vi "Motion Profile Generator Jerk Limited.vi"() -> ()   [LabVIEW 2016]
panel:
  out "Final Position":dbl=202.3936431884765
  out "acceleration rotations/sec^2":dbl[](array[numeric])=[0.0, 2.2612551610354346, 4.522510322070869, 6.783765483106304, 9.045020644141736, 11.30627580517718, 13.567530966212601, 15.828786127248051, 18.090041288283476, 20.351296449318905, 22.612551610354323, 24.873806771389795, 27.135061932425213, 29.396317093460667, 31.657572254496067, 33.91882741553147, 36.18008257656694, 38.441337737602375, 40.702592898637846, 42.96384805967321, 45.22510322070865, 47.48635838174408, 49.74761354277966, 52.008868703814954, 54.27012386485039, 56.531379025885826, 58.79263418692133, 58.79263418692119, 56.531379025885826, 54.27012386485046, 52.0088687038151, 49.74761354277945, 47.48635838174408, 45.22510322070886, 42.96384805967321, 40.702592898637704, 38.44133773760234, 36.180082576567116, 33.918827415531325, 31.657572254496245, 29.396317093460596, 27.13506193242523, 24.873806771389866, 22.612551610354217, 20.351296449319136, 18.090041288283203, 15.828786127248122, 13.567530966212757, 11.306275805177393, 9.045020644141744, 6.7837654831060945, 4.522510322071014, 0.0, -4.522510322071014, -6.7837654831060945, -9.045020644141744, -11.306275805177393, -13.567530966212473, -15.828786127248122, -18.090041288283203, -20.351296449319136, -22.612551610353933, -24.87380677139015, -27.135061932424946, -29.39631709346088, -31.65757225449596, -33.91882741553161, -36.18008257656669, -38.44133773760248, -40.70259289863799, -42.96384805967307, -45.22510322070872, -47.48635838174408, -49.74761354277959, -52.00886870381467, -54.2701238648506, -56.531379025885826, -58.792634186921475, -58.79263418692119, -56.531379025885684, -54.27012386485046, -52.008868703815025, -49.74761354277952, -47.486358381744154, -45.22510322070872, -42.96384805967335, -40.702592898637775, -38.44133773760241, -36.18008257656694, -33.91882741553154, -31.657572254496102, -29.396317093460667, -27.13506193242525, -24.873806771389813, -22.61255161035436, -20.351296449318923, -18.090041288283523, -15.82878612724806, -13.567530966212637, -11.306275805177197, -9.04502064414177, -6.783765483106331, -4.522510322070896, -2.261255161035462, -2.774099786489076e-14]
  out "Position rotations":dbl[](array[numeric])=[0.0, 0.002826568951294293, 0.014132844756471467, 0.039571965318120114, 0.08479706853882882, 0.15546129232118616, 0.2572177745677807, 0.3957196531812011, 0.5766200660640359, 0.8055721511188737, 1.088229046248303, 1.4302438893549125, 1.8372698183412908, 2.314959971110026, 2.8689674855637075, 3.5049454996049234, 4.2285471511362624, 5.045425578060313, 5.961233918279664, 6.981625309696904, 8.11225289021462, 9.358769797735404, 10.72682917016184, 12.222084145396522, 13.850187861342034, 15.616793455900966, 17.52755406697591, 19.585296263518153, 21.787193476576405, 24.12759256824808, 26.600840400630585, 29.201283835821336, 31.92326973591774, 34.76114496301721, 37.70925637921716, 40.761950846614994, 43.91357522730813, 47.158476383393975, 50.491001176969945, 53.90549647013345, 57.396309124981904, 60.95778600361271, 64.58427396812328, 68.27011988061105, 72.00967060317339, 75.79727299790774, 79.6272739269115, 83.4940202522821, 87.39185883611692, 91.31513654051341, 95.25820022756895, 99.21539675938097, 103.17824642909557, 107.13544296090758, 111.07850664796312, 115.0017843523596, 118.89962293619443, 122.76636926156503, 126.5963701905688, 130.38397258530316, 134.1235233078655, 137.80936922035326, 141.43585718486383, 144.99733406349463, 148.48814671834307, 151.90264201150657, 155.23516680508254, 158.4800679611684, 161.63169234186154, 164.68438680925937, 167.6324982254593, 170.47037345255876, 173.19235935265516, 175.79280278784591, 178.2660506202284, 180.6064497119001, 182.80834692495836, 184.8660891215006, 186.77684973257556, 188.5434553271345, 190.17155904308, 191.66681401831468, 193.03487339074113, 194.2813902982619, 195.4120178787796, 196.43240927019684, 197.34821761041619, 198.16509603734025, 198.8886976888716, 199.52467570291282, 200.0786832173665, 200.55637337013522, 200.9633992991216, 201.3054141422282, 201.58807103735762, 201.81702312241245, 201.99792353529529, 202.1364254139087, 202.2381818961553, 202.30884611993767, 202.35407122315837, 202.37951034372003, 202.3908166195252, 202.3936431884765, 202.3936431884765]
  out "velocity rotations/sec":dbl[](array[numeric])=[0.0, 0.11306275805177173, 0.3391882741553152, 0.6783765483106304, 1.1306275805177173, 1.6959413707765763, 2.3743179190872064, 3.165757225449609, 4.070259289863783, 5.087824112329728, 6.218451692847444, 7.462142031416934, 8.818895128038195, 10.288710982711228, 11.871589595436031, 13.567530966212605, 15.376535095040952, 17.29860198192107, 19.333731626852963, 21.481924029836623, 23.743179190872056, 26.11749710995926, 28.604877787098243, 31.20532122228899, 33.91882741553151, 36.7453963668258, 39.68502807617187, 42.62465978551793, 45.45122873681222, 48.16473493005474, 50.7651783652455, 53.25255904238447, 55.62687696147167, 57.888132122507116, 60.03632452549078, 62.07145417042266, 63.99352105730278, 65.80252518613113, 67.4984665569077, 69.08134516963251, 70.55116102430554, 71.9079141209268, 73.1516044594963, 74.28223204001401, 75.29979686247997, 76.20429892689413, 76.99573823325653, 77.67411478156717, 78.23942857182604, 78.69167960403313, 79.03086787818843, 79.25699339429198, 79.25699339429198, 79.03086787818843, 78.69167960403313, 78.23942857182604, 77.67411478156717, 76.99573823325655, 76.20429892689414, 75.29979686247998, 74.28223204001402, 73.15160445949633, 71.90791412092682, 70.55116102430557, 69.08134516963253, 67.49846655690773, 65.80252518613115, 63.993521057302814, 62.07145417042269, 60.03632452549079, 57.88813212250714, 55.6268769614717, 53.2525590423845, 50.76517836524552, 48.164734930054784, 45.451228736812254, 42.62465978551796, 39.68502807617189, 36.74539636682583, 33.918827415531545, 31.205321222289022, 28.60487778709827, 26.117497109959295, 23.743179190872088, 21.48192402983665, 19.333731626852984, 17.298601981921095, 15.376535095040975, 13.567530966212628, 11.87158959543605, 10.288710982711246, 8.818895128038212, 7.46214203141695, 6.218451692847459, 5.087824112329741, 4.070259289863795, 3.165757225449619, 2.374317919087216, 1.6959413707765842, 1.1306275805177244, 0.6783765483106359, 0.3391882741553193, 0.1130627580517745, 1.3870498932445381e-15, 0.0]
  out "XY Graph":cluster{dbl[], dbl[]}[](graph)=[{[0.0, 0.05, 0.1, 0.15000000000000002, 0.2, 0.25, 0.30000000000000004, 0.35000000000000003, 0.4, 0.45, 0.5, 0.55, 0.6000000000000001, 0.65, 0.7000000000000001, 0.75, 0.8, 0.8500000000000001, 0.9, 0.9500000000000001, 1.0, 1.05, 1.1, 1.1500000000000001, 1.2000000000000002, 1.25, 1.3, 1.35, 1.4000000000000001, 1.4500000000000002, 1.5, 1.55, 1.6, 1.6500000000000001, 1.7000000000000002, 1.75, 1.8, 1.85, 1.9000000000000001, 1.9500000000000002, 2.0, 2.0500000000000003, 2.1, 2.15, 2.2, 2.25, 2.3000000000000003, 2.35, 2.4000000000000004, 2.45, 2.5, 2.5500000000000003, 2.6, 2.6500000000000004, 2.7, 2.75, 2.8000000000000003, 2.85, 2.9000000000000004, 2.95, 3.0, 3.0500000000000003, 3.1, 3.1500000000000004, 3.2, 3.25, 3.3000000000000003, 3.35, 3.4000000000000004, 3.45, 3.5, 3.5500000000000003, 3.6, 3.6500000000000004, 3.7, 3.75, 3.8000000000000003, 3.85, 3.9000000000000004, 3.95, 4.0, 4.05, 4.1000000000000005, 4.15, 4.2, 4.25, 4.3, 4.3500000000000005, 4.4, 4.45, 4.5, 4.55, 4.6000000000000005, 4.65, 4.7, 4.75, 4.800000000000001, 4.8500000000000005, 4.9, 4.95, 5.0, 5.050000000000001, 5.1000000000000005, 5.15, 5.2], [0.0, 0.11306275805177173, 0.3391882741553152, 0.6783765483106304, 1.1306275805177173, 1.6959413707765763, 2.3743179190872064, 3.165757225449609, 4.070259289863783, 5.087824112329728, 6.218451692847444, 7.462142031416934, 8.818895128038195, 10.288710982711228, 11.871589595436031, 13.567530966212605, 15.376535095040952, 17.29860198192107, 19.333731626852963, 21.481924029836623, 23.743179190872056, 26.11749710995926, 28.604877787098243, 31.20532122228899, 33.91882741553151, 36.7453963668258, 39.68502807617187, 42.62465978551793, 45.45122873681222, 48.16473493005474, 50.7651783652455, 53.25255904238447, 55.62687696147167, 57.888132122507116, 60.03632452549078, 62.07145417042266, 63.99352105730278, 65.80252518613113, 67.4984665569077, 69.08134516963251, 70.55116102430554, 71.9079141209268, 73.1516044594963, 74.28223204001401, 75.29979686247997, 76.20429892689413, 76.99573823325653, 77.67411478156717, 78.23942857182604, 78.69167960403313, 79.03086787818843, 79.25699339429198, 79.25699339429198, 79.03086787818843, 78.69167960403313, 78.23942857182604, 77.67411478156717, 76.99573823325655, 76.20429892689414, 75.29979686247998, 74.28223204001402, 73.15160445949633, 71.90791412092682, 70.55116102430557, 69.08134516963253, 67.49846655690773, 65.80252518613115, 63.993521057302814, 62.07145417042269, 60.03632452549079, 57.88813212250714, 55.6268769614717, 53.2525590423845, 50.76517836524552, 48.164734930054784, 45.451228736812254, 42.62465978551796, 39.68502807617189, 36.74539636682583, 33.918827415531545, 31.205321222289022, 28.60487778709827, 26.117497109959295, 23.743179190872088, 21.48192402983665, 19.333731626852984, 17.298601981921095, 15.376535095040975, 13.567530966212628, 11.87158959543605, 10.288710982711246, 8.818895128038212, 7.46214203141695, 6.218451692847459, 5.087824112329741, 4.070259289863795, 3.165757225449619, 2.374317919087216, 1.6959413707765842, 1.1306275805177244, 0.6783765483106359, 0.3391882741553193, 0.1130627580517745, 1.3870498932445381e-15, 0.0]}, {[0.0, 0.05, 0.1, 0.15000000000000002, 0.2, 0.25, 0.30000000000000004, 0.35000000000000003, 0.4, 0.45, 0.5, 0.55, 0.6000000000000001, 0.65, 0.7000000000000001, 0.75, 0.8, 0.8500000000000001, 0.9, 0.9500000000000001, 1.0, 1.05, 1.1, 1.1500000000000001, 1.2000000000000002, 1.25, 1.3, 1.35, 1.4000000000000001, 1.4500000000000002, 1.5, 1.55, 1.6, 1.6500000000000001, 1.7000000000000002, 1.75, 1.8, 1.85, 1.9000000000000001, 1.9500000000000002, 2.0, 2.0500000000000003, 2.1, 2.15, 2.2, 2.25, 2.3000000000000003, 2.35, 2.4000000000000004, 2.45, 2.5, 2.5500000000000003, 2.6, 2.6500000000000004, 2.7, 2.75, 2.8000000000000003, 2.85, 2.9000000000000004, 2.95, 3.0, 3.0500000000000003, 3.1, 3.1500000000000004, 3.2, 3.25, 3.3000000000000003, 3.35, 3.4000000000000004, 3.45, 3.5, 3.5500000000000003, 3.6, 3.6500000000000004, 3.7, 3.75, 3.8000000000000003, 3.85, 3.9000000000000004, 3.95, 4.0, 4.05, 4.1000000000000005, 4.15, 4.2, 4.25, 4.3, 4.3500000000000005, 4.4, 4.45, 4.5, 4.55, 4.6000000000000005, 4.65, 4.7, 4.75, 4.800000000000001, 4.8500000000000005, 4.9, 4.95, 5.0, 5.050000000000001, 5.1000000000000005, 5.15, 5.2], [0.0, 0.002826568951294293, 0.014132844756471467, 0.039571965318120114, 0.08479706853882882, 0.15546129232118616, 0.2572177745677807, 0.3957196531812011, 0.5766200660640359, 0.8055721511188737, 1.088229046248303, 1.4302438893549125, 1.8372698183412908, 2.314959971110026, 2.8689674855637075, 3.5049454996049234, 4.2285471511362624, 5.045425578060313, 5.961233918279664, 6.981625309696904, 8.11225289021462, 9.358769797735404, 10.72682917016184, 12.222084145396522, 13.850187861342034, 15.616793455900966, 17.52755406697591, 19.585296263518153, 21.787193476576405, 24.12759256824808, 26.600840400630585, 29.201283835821336, 31.92326973591774, 34.76114496301721, 37.70925637921716, 40.761950846614994, 43.91357522730813, 47.158476383393975, 50.491001176969945, 53.90549647013345, 57.396309124981904, 60.95778600361271, 64.58427396812328, 68.27011988061105, 72.00967060317339, 75.79727299790774, 79.6272739269115, 83.4940202522821, 87.39185883611692, 91.31513654051341, 95.25820022756895, 99.21539675938097, 103.17824642909557, 107.13544296090758, 111.07850664796312, 115.0017843523596, 118.89962293619443, 122.76636926156503, 126.5963701905688, 130.38397258530316, 134.1235233078655, 137.80936922035326, 141.43585718486383, 144.99733406349463, 148.48814671834307, 151.90264201150657, 155.23516680508254, 158.4800679611684, 161.63169234186154, 164.68438680925937, 167.6324982254593, 170.47037345255876, 173.19235935265516, 175.79280278784591, 178.2660506202284, 180.6064497119001, 182.80834692495836, 184.8660891215006, 186.77684973257556, 188.5434553271345, 190.17155904308, 191.66681401831468, 193.03487339074113, 194.2813902982619, 195.4120178787796, 196.43240927019684, 197.34821761041619, 198.16509603734025, 198.8886976888716, 199.52467570291282, 200.0786832173665, 200.55637337013522, 200.9633992991216, 201.3054141422282, 201.58807103735762, 201.81702312241245, 201.99792353529529, 202.1364254139087, 202.2381818961553, 202.30884611993767, 202.35407122315837, 202.37951034372003, 202.3908166195252, 202.3936431884765, 202.3936431884765]}, {[0.0, 0.05, 0.1, 0.15000000000000002, 0.2, 0.25, 0.30000000000000004, 0.35000000000000003, 0.4, 0.45, 0.5, 0.55, 0.6000000000000001, 0.65, 0.7000000000000001, 0.75, 0.8, 0.8500000000000001, 0.9, 0.9500000000000001, 1.0, 1.05, 1.1, 1.1500000000000001, 1.2000000000000002, 1.25, 1.3, 1.35, 1.4000000000000001, 1.4500000000000002, 1.5, 1.55, 1.6, 1.6500000000000001, 1.7000000000000002, 1.75, 1.8, 1.85, 1.9000000000000001, 1.9500000000000002, 2.0, 2.0500000000000003, 2.1, 2.15, 2.2, 2.25, 2.3000000000000003, 2.35, 2.4000000000000004, 2.45, 2.5, 2.5500000000000003, 2.6, 2.6500000000000004, 2.7, 2.75, 2.8000000000000003, 2.85, 2.9000000000000004, 2.95, 3.0, 3.0500000000000003, 3.1, 3.1500000000000004, 3.2, 3.25, 3.3000000000000003, 3.35, 3.4000000000000004, 3.45, 3.5, 3.5500000000000003, 3.6, 3.6500000000000004, 3.7, 3.75, 3.8000000000000003, 3.85, 3.9000000000000004, 3.95, 4.0, 4.05, 4.1000000000000005, 4.15, 4.2, 4.25, 4.3, 4.3500000000000005, 4.4, 4.45, 4.5, 4.55, 4.6000000000000005, 4.65, 4.7, 4.75, 4.800000000000001, 4.8500000000000005, 4.9, 4.95, 5.0, 5.050000000000001, 5.1000000000000005, 5.15, 5.2], [0.0, 2.2612551610354346, 4.522510322070869, 6.783765483106304, 9.045020644141736, 11.30627580517718, 13.567530966212601, 15.828786127248051, 18.090041288283476, 20.351296449318905, 22.612551610354323, 24.873806771389795, 27.135061932425213, 29.396317093460667, 31.657572254496067, 33.91882741553147, 36.18008257656694, 38.441337737602375, 40.702592898637846, 42.96384805967321, 45.22510322070865, 47.48635838174408, 49.74761354277966, 52.008868703814954, 54.27012386485039, 56.531379025885826, 58.79263418692133, 58.79263418692119, 56.531379025885826, 54.27012386485046, 52.0088687038151, 49.74761354277945, 47.48635838174408, 45.22510322070886, 42.96384805967321, 40.702592898637704, 38.44133773760234, 36.180082576567116, 33.918827415531325, 31.657572254496245, 29.396317093460596, 27.13506193242523, 24.873806771389866, 22.612551610354217, 20.351296449319136, 18.090041288283203, 15.828786127248122, 13.567530966212757, 11.306275805177393, 9.045020644141744, 6.7837654831060945, 4.522510322071014, 0.0, -4.522510322071014, -6.7837654831060945, -9.045020644141744, -11.306275805177393, -13.567530966212473, -15.828786127248122, -18.090041288283203, -20.351296449319136, -22.612551610353933, -24.87380677139015, -27.135061932424946, -29.39631709346088, -31.65757225449596, -33.91882741553161, -36.18008257656669, -38.44133773760248, -40.70259289863799, -42.96384805967307, -45.22510322070872, -47.48635838174408, -49.74761354277959, -52.00886870381467, -54.2701238648506, -56.531379025885826, -58.792634186921475, -58.79263418692119, -56.531379025885684, -54.27012386485046, -52.008868703815025, -49.74761354277952, -47.486358381744154, -45.22510322070872, -42.96384805967335, -40.702592898637775, -38.44133773760241, -36.18008257656694, -33.91882741553154, -31.657572254496102, -29.396317093460667, -27.13506193242525, -24.873806771389813, -22.61255161035436, -20.351296449318923, -18.090041288283523, -15.82878612724806, -13.567530966212637, -11.306275805177197, -9.04502064414177, -6.783765483106331, -4.522510322070896, -2.261255161035462, -2.774099786489076e-14]}]
  in  "ms per frame":dbl=20.0
  in  "Max Jerk (In/sec^3)":dbl=50.0
  in  "Max Acceleration (In/sec^2)":dbl=100.0
  in  "Inches to Travel":dbl=200.0
  in  "Max Speed (In/sec)":dbl=100.0
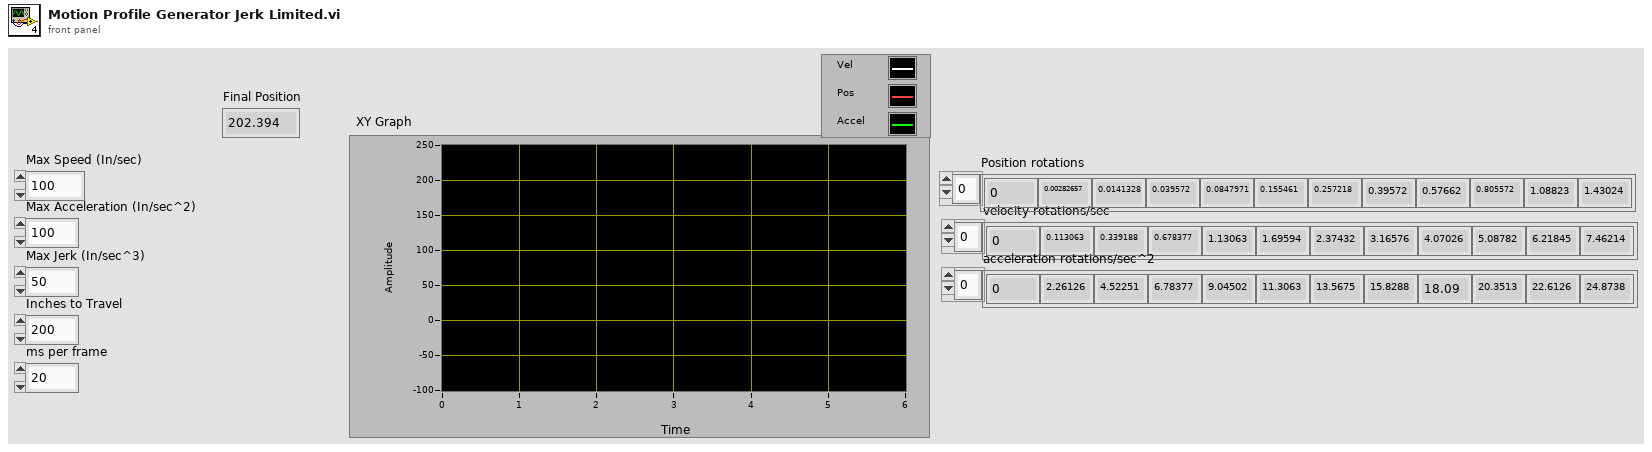
[diagram p1: front panel]
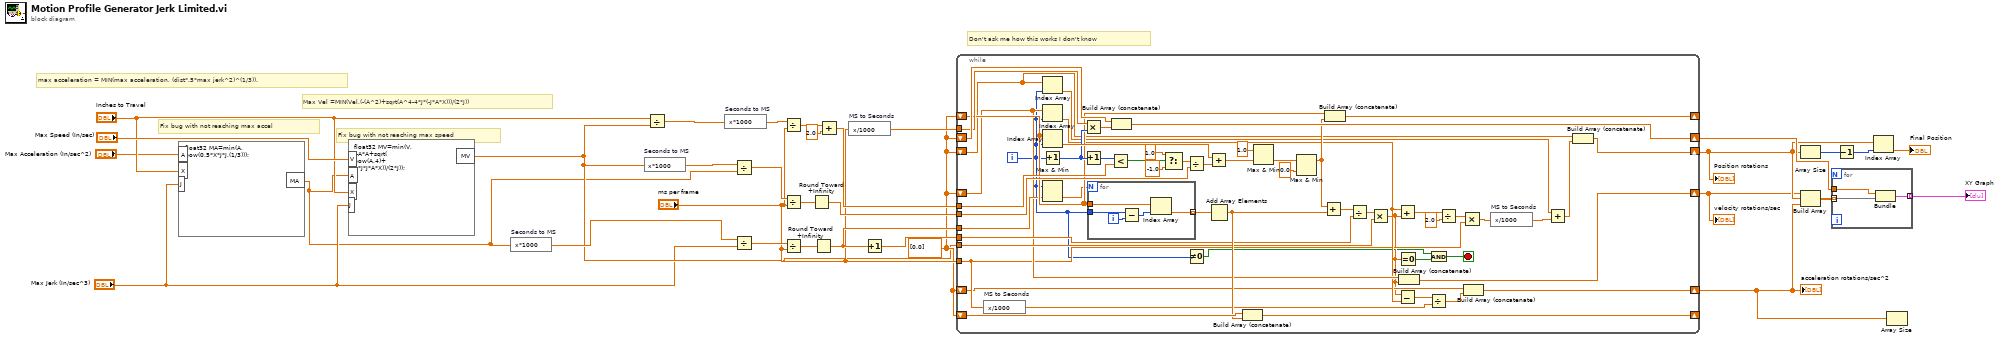
[diagram p0: block diagram]
diagram:
  w16 = dbl[] [0.0]
  # "Fix bug with not reaching max accel"
  # "max acceleration = MIN(max acceleration, (dist*.5*max jerk^2)^(1/3))."
  # "Don't ask me how this works I don't know"
  # "Fix bug with not reaching max speed"
  # "Max Vel =MIN(Vel,(-(A^2)+sqrt(A^4-4*J*(-J*A*X)))/(2*J))"
  n1 = formula code="float32 MA=min(A,\npow(0.5*X*J*J,(1/3)));"("A"="Max Acceleration (In/sec^2)", "X"="Inches to Travel", "J"="Max Jerk (In/sec^3)") -> ("MA"=w2:sgl)
  n2 = formula code="float32 MV=min(V,\n(-A*A+sqrt(\npow(A,4)+\n4*J*J*A*X))/(2*J));"("V"="Max Speed (In/sec)", "A"=w2, "X"="Inches to Travel", "J"="Max Jerk (In/sec^3)") -> ("MV"=w7:sgl)
  n3 = expression code="x*1000" "Seconds to MS"(w2) -> (w31:sgl)
  n4 = expression code="x*1000" "Seconds to MS"(w7) -> (w30:sgl)
  n5 = Divide(x="Inches to Travel", y=w7) -> (x/y=w29:dbl)
  n6 = expression code="x*1000" "Seconds to MS"(w29) -> (w28:dbl)
  n7 = Divide(x=w30, y=w2) -> (x/y=w24:sgl)
  n8 = Divide(x=w31, y="Max Jerk (In/sec^3)") -> (x/y=w21:dbl)
  n9 = Divide(x=w28, y="ms per frame") -> (x/y=w27:dbl)
  n10 = Divide(x=w24, y="ms per frame") -> (x/y=w23:dbl)
  n11 = Divide(x=w21, y="ms per frame") -> (x/y=w20:dbl)
  n12 = Round Toward +Infinity(x=w23) -> (ceil(x): smallest int >= x=w22:dbl)
  n13 = Round Toward +Infinity(x=w20) -> (ceil(x): smallest int >= x=w19:dbl)
  n14 = Add(x=w27, y=2.0) -> (x+y=w25:dbl)
  n15 = expression code="x/1000" "MS to Seconds"("ms per frame") -> (w32:dbl)
  n16 = Increment(x=w19) -> (x+1=w18:dbl)
  n17 = while {
    shift-right: [w85] -> w14
    shift-left: w16 -> [w86]
    tunnel: w32 -> [w84]
    tunnel: w25 -> [w82]
    shift-right: [w68] -> _
    shift-left: w16 -> [w67]
    tunnel: w22 -> [w74]
    tunnel: w19 -> [w65]
    shift-right: [w62] -> _
    shift-left: w16 -> [w63]
    tunnel: w18 -> [w58]
    tunnel: w7 -> [w56]
    shift-right: [w55] -> w8
    shift-left: w16 -> [w53]
    shift-right: [w54] -> w9
    shift-left: w16 -> [w47]
    tunnel: "ms per frame" -> [w41]
    shift-right: [w39] -> w1
    shift-left: w16 -> [w38]
    i -> [w37]
    stop <- w33 stop-if-true
    n18 = expression code="x/1000" "MS to Seconds"(w41) -> (w42:dbl)
    n19 = Index Array(array=w47, index=w37) -> (element=w46:dbl)
    n20 = Index Array(array=w53, index=w37) -> (element=w44:dbl)
    n21 = Index Array(array=w67, index=w37) -> (element=w72:dbl)
    n22 = Increment(x=w37) -> (x+1=w70:i32)
    n23 = Max & Min(x=w37, y=w65) -> (min(x,y)=w64:dbl)  [unwired: 1 out]
    n24 = Multiply(x=w84, y=w70) -> (x*y=w83:dbl)
    n25 = Increment(x=w70) -> (x+1=w71:i32)
    n26 = for {
      N: w64 -> [_]
      tunnel: w37 -> [w90]
      tunnel: w67 -> [w88]
      tunnel: [w87] -> w66 mode=indexing
      i -> [w91]
      n27 = Subtract(x=w90, y=w91) -> (x-y=w89:i32)
      n28 = Index Array(array=w88, index=w89) -> (element=w87:dbl)
    }
    n29 = Less?(x=w71, y=w82) -> (x < y?=w78:bool)
    n30 = Build Array (concatenate)(w86, w83) -> (w85:dbl[])
    n31 = Select(t=1.0, s=w78, f=-1.0) -> (s? t:f=w75:dbl)
    n32 = Divide(x=w75, y=w74) -> (x/y=w73:dbl)
    n33 = Not Equal To 0?(x=w37) -> (x != 0?=w34:bool)
    n34 = Add(x=w72, y=w73) -> (x+y=w69:dbl)
    n35 = Add Array Elements(numeric array=w66) -> (sum=w61:dbl)
    n36 = Build Array (concatenate)(w63, w61) -> (w62:dbl[])
    n37 = Max & Min(x=1.0, y=w69) -> (min(x,y)=w80:dbl)  [unwired: 1 out]
    n38 = Max & Min(x=w80, y=0.0) -> (max(x,y)=w60:dbl)  [unwired: 1 out]
    n39 = Add(x=w60, y=w61) -> (x+y=w59:dbl)
    n40 = Build Array (concatenate)(w67, w60) -> (w68:dbl[])
    n41 = Divide(x=w59, y=w58) -> (x/y=w57:dbl)
    n42 = Multiply(x=w57, y=w56) -> (x*y=w36:dbl)
    n43 = Add(x=w44, y=w36) -> (x+y=w52:dbl)
    n44 = Subtract(x=w36, y=w44) -> (x-y=w43:dbl)
    n45 = Equal To 0?(x=w36) -> (x = 0?=w35:bool)
    n46 = Build Array (concatenate)(w53, w36) -> (w55:dbl[])
    n47 = Divide(x=w43, y=w42) -> (x/y=w40:dbl)
    n48 = And(x=w34, y=w35) -> (x .and. y?=w33:bool)
    n49 = Divide(x=w52, y=2.0) -> (x/y=w50:dbl)
    n50 = Multiply(x=w50, y=w41) -> (x*y=w49:dbl)
    n51 = Build Array (concatenate)(w38, w40) -> (w39:dbl[])
    n52 = expression code="x/1000" "MS to Seconds"(w49) -> (w48:dbl)
    n53 = Add(x=w46, y=w48) -> (x+y=w45:dbl)
    n54 = Build Array (concatenate)(w47, w45) -> (w54:dbl[])
  }
  "velocity rotations/sec" <- w8
  "Position rotations" <- w9
  "acceleration rotations/sec^2" <- w1
  n55 = Array Size(array=w9) -> (size(s)=w12:i32)
  n56 = Build Array(w8, w9, w1) -> (w15:dbl[][])
  n57 = for {
    tunnel: w15 -> [w94] mode=indexing
    tunnel: w14 -> [w93]
    tunnel: [w92] -> w13 mode=indexing
    n58 = Bundle(w93, w94) -> (w92:cluster{dbl[], dbl[]})  [unwired: 1 in]
  }
  "XY Graph" <- w13
  n59 = Decrement(x=w12) -> (x-1=w11:i32)
  n60 = Index Array(array=w9, index=w11) -> (element=→"Final Position":dbl)
  n61 = Array Size(array=w1) -> ()  [unwired: 1 out]
